vi "Laser line to DO number.vi"(8 "error in (no error)":errorcluster, 10 "Wavelength":T1 items=["Blind"=10, "405nm"=0, "445nm"=5, "491nm"=1, "515nm"=2, "488nm"=3], 11 "AOTF in":refnum<class "AOTF.lvclass">) -> (0 "error out":errorcluster, 2 "DO number":bool[](array[boolean]), 3 "AOTF out":refnum<class "AOTF.lvclass">)   [LabVIEW 2012, in "AOTF.lvclass"]
uses:
  AOTF.lvclass
  Controls/laser line ring.ctl
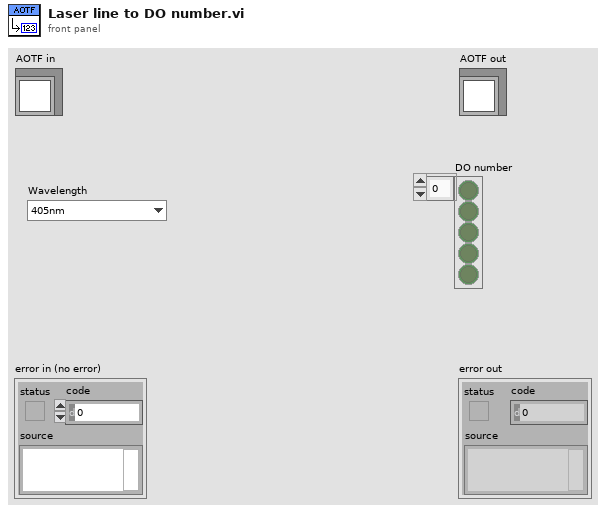
[diagram p1: front panel]
types:
  T1 = typedef "AOTF.lvclass/laser line ring.ctl" = u8
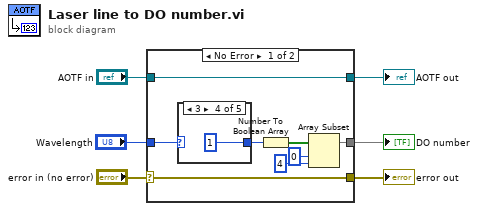
[diagram p0: block diagram]
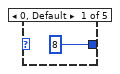
[diagram p2: hidden frame]
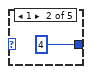
[diagram p3: hidden frame]
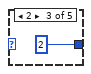
[diagram p4: hidden frame]
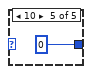
[diagram p5: hidden frame]
diagram:
  n1 = case shown="No Error" "error in (no error)" {
    selector: "error in (no error)" -> [w13 w21]
    tunnel: [w13 w21] -> w5
    tunnel: [w14 w20] -> w3
    tunnel: "AOTF in" -> [w14 w20]
    tunnel: "Wavelength" -> [w12 _]
    tunnel: [w9 _] -> w1
    frame No Error {
      n2 = case shown="3" w12 {
        tunnel: [u32 8 ("DO number") u32 4 ("DO number") u32 2 ("DO number") u32 1 ("DO number") u32 0 ("DO number")] -> w11
        frame 0, Default {
        }
        frame 1 {
        }
        frame 2 {
        }
        frame 3 {
        }
        frame 10 {
        }
      }
      n3 = Number To Boolean Array(number=w11) -> (Boolean array=w10:bool[])
      n4 = Array Subset(array=w10, index=0, length=4) -> (w9:bool[])
    }
    frame Error {
    }
  }
  "error out" <- w5
  "AOTF out" <- w3
  "DO number" <- w1
